vi "Get MListbox Ref.vi"(8 "error in (no error)":errorcluster, 11 "Multicolumn ListBox in":refnum<class "Multicolumn ListBox.lvclass">) -> (0 "error out":errorcluster, 2 "MListbox Ref":refnum<vi>, 3 "Multicolumn ListBox out":refnum<class "Multicolumn ListBox.lvclass">)   [LabVIEW 2018, in "Multicolumn ListBox.lvclass"]
uses:
  Multicolumn ListBox.lvclass
  Multicolumn ListBox.lvclass/Multicolumn ListBox.ctl
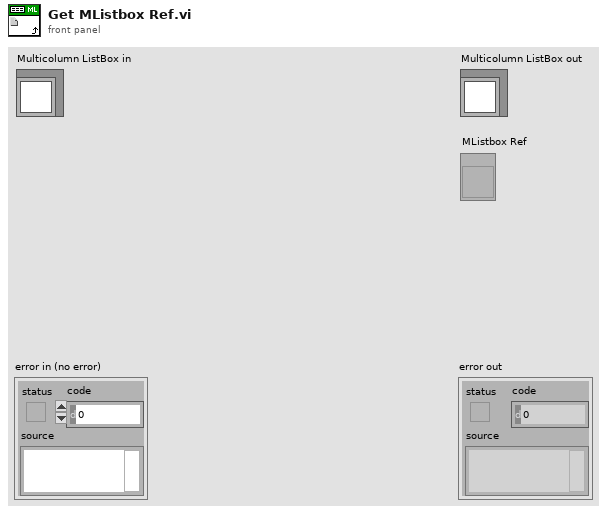
[diagram p1: front panel]
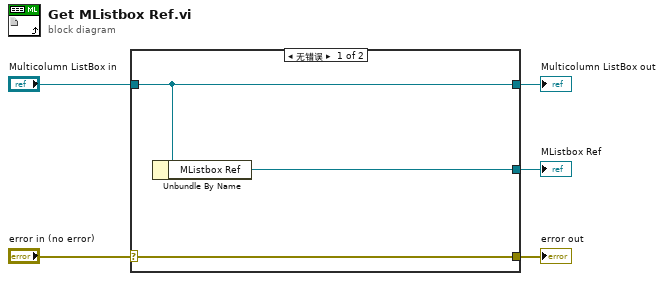
[diagram p0: block diagram]
diagram:
  n1 = case shown="无错误" "error in (no error)" {
    selector: "error in (no error)" -> [w8 w9]
    tunnel: [w8 w9] -> w4
    tunnel: [w7 w10] -> w2
    tunnel: "Multicolumn ListBox in" -> [w7 w10]
    tunnel: [w6 _] -> w1
    frame No Error {
      n2 = Unbundle By Name(w7) -> ("MListbox Ref"=w6:refnum<vi>)
    }
    frame Error {
    }
  }
  "error out" <- w4
  "Multicolumn ListBox out" <- w2
  "MListbox Ref" <- w1
